vi "read_temp_registers.vi"(0 "Serial sessions":refnum<class "MB_Master_Serial.lvclass">[](array[class]), 3 "error in":errorcluster) -> (7 "Serial out":refnum<class "MB_Master_Serial.lvclass">[](array[class]), 8 "Array of temperatures":dbl[][](array[numeric]), 10 "error out":errorcluster)   [LabVIEW 2017, in "Akwizycja.lvlib"]
uses:
  Akwizycja.lvlib
  <vilib>/Plasmionique/MB Master/MB_Master_Serial/MB_Master_Serial.lvclass
  D:/Program Files (x86)/National Instruments/LabVIEW 2017/vi.lib/Plasmionique/MB Master/MB_Master/MB_Master.lvclass
  <vilib>/Plasmionique/MB Master/MB Master.lvlib
panel:
  in  "Array 2":dbl[][](array[numeric])
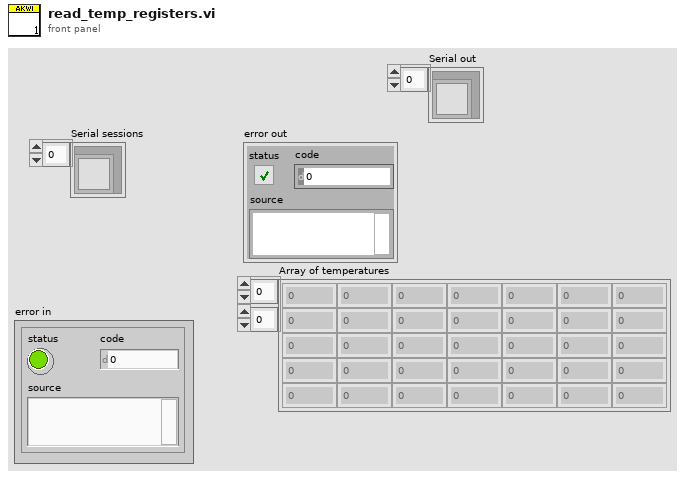
[diagram p1: front panel]
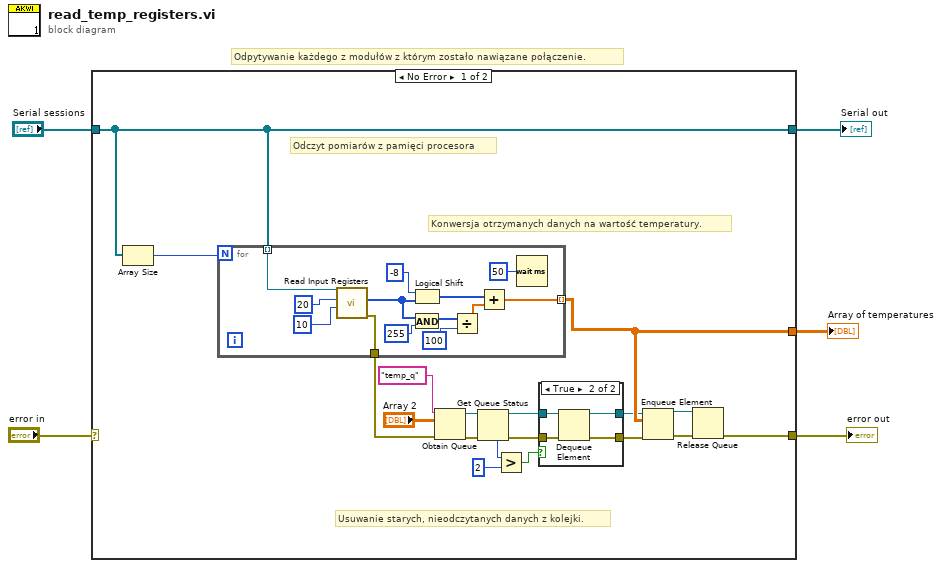
[diagram p0: block diagram]
diagram:
  # "Odpytywanie każdego z modułów z którym zostało nawiązane połączenie."
  n1 = case shown="No Error" "error in" {
    selector: "error in" -> [_ w44]
    tunnel: [w19 w44] -> w5
    tunnel: "Serial sessions" -> [w6 w43]
    tunnel: [w16 _] -> w2
    tunnel: [w6 w43] -> w1
    frame No Error {
      # "Odczyt pomiarów z pamięci procesora"
      # "Konwersja otrzymanych danych na wartość temperatury."
      # "Usuwanie starych, nieodczytanych danych z kolejki."
      n2 = Array Size(array=w6) -> (size(s)=w17:i32)
      n3 = for {
        N: w17 -> [_]
        tunnel: [w40] -> w23
        tunnel: w6 -> [w31] mode=indexing
        tunnel: [w32] -> w16 mode=indexing
        n4 = call <vilib>:"Read Input Registers.vi"("quantity"=u16 10, "starting address"=u16 20, "MB session in"=w31) -> ("error out"=w40:errorcluster, "Registers"=w37:u16[])  [unwired: 6 in, 1 out]
        n5 = Logical Shift(y=i16 -8, x=w37) -> (x << y=w36:u16[])
        n6 = And(x=w37, y=255) -> (x .and. y?=w35:i32[])
        n7 = Divide(x=w35, y=100) -> (x/y=w33:dbl[])
        n8 = Add(x=w36, y=w33) -> (x+y=w32:dbl[])
        n9 = Wait (ms)(milliseconds to wait=u32 50) -> ()  [unwired: 1 out]
      }
      n10 = Obtain Queue(name (unnamed)="temp_q", element data type="Array 2", error in (no error)=w23) -> (queue out=w8:refnum<queue>, error out=w7:errorcluster)  [unwired: 2 in, 1 out]
      n11 = Get Queue Status(queue=w8, error in (no error)=w7) -> (queue out=w12:refnum<queue>, error out=w15:errorcluster, # elements in queue=w14:i32)  [unwired: 1 in, 5 out]
      n12 = Greater?(x=w14, y=2) -> (0:w11:bool)
      n13 = case shown="True" w11 {
        tunnel: w15 -> [w24 w29]
        tunnel: w12 -> [w25 w28]
        tunnel: [w25 w27] -> w10
        tunnel: [w24 w26] -> w9
        frame False {
        }
        frame True {
          n14 = Dequeue Element(queue=w28, error in (no error)=w29) -> (queue out=w27:refnum<queue>, error out=w26:errorcluster)  [unwired: 1 in, 2 out]
        }
      }
      n15 = Enqueue Element(queue=w10, element=w16, error in (no error)=w9) -> (queue out=w21:refnum<queue>, error out=w20:errorcluster)  [unwired: 1 in, 1 out]
      n16 = Release Queue(queue=w21, error in (no error)=w20) -> (error out=w19:errorcluster)  [unwired: 1 in, 2 out]
    }
    frame Error {
    }
  }
  "error out" <- w5
  "Array of temperatures" <- w2
  "Serial out" <- w1
